vi "Get Log State.vi"(8 "error in (no error)":errorcluster, 10 "Buffer Name (defbuffer1)":string="defbuffer1", 11 "VISA resource name":refnum<visa-resource-name>) -> (0 "error out":errorcluster, 2 "Logging Enabled?":bool, 3 "VISA resource name out":refnum<visa-resource-name>)   [LabVIEW 2022 SP3, in "Keithley 2450.lvlib"]
doc: "This returns whether the reading buffer logs informational events."
uses:
  Keithley 2450.lvlib
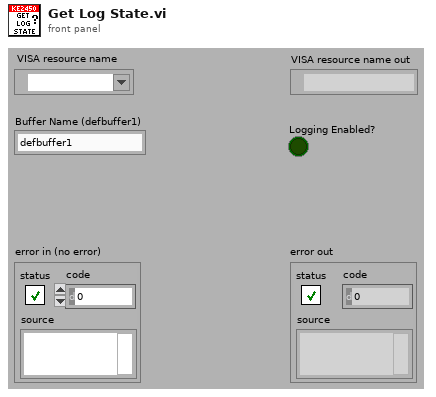
[diagram p1: front panel]
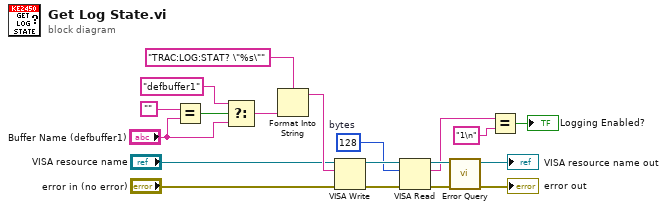
[diagram p0: block diagram]
diagram:
  w4 = u32 128  # bytes
  n1 = Equal?(x="", y="Buffer Name (defbuffer1)") -> (x = y?=w12:bool)
  n2 = Select(t="defbuffer1", s=w12, f="Buffer Name (defbuffer1)") -> (s? t:f=w9:string)
  n3 = Format Into String(format string="TRAC:LOG:STAT? \"%s\"", w9) -> (resulting string=w16:string)  [unwired: 2 in, 1 out]
  n4 = VISA Write(VISA resource name="VISA resource name", write buffer=w16, error in (no error)="error in (no error)") -> (VISA resource name out=w8:refnum<visa-resource-name>, error out=w6:errorcluster)  [unwired: 1 out]
  n5 = VISA Read(VISA resource name=w8, byte count=w4, error in (no error)=w6) -> (VISA resource name out=w7:refnum<visa-resource-name>, read buffer=w1:string, error out=w5:errorcluster)  [unwired: 1 out]
  n6 = call "Error Query.vi"("error in (no error)"=w5, "VISA resource name"=w7) -> ("error out"=→"error out":errorcluster, "VISA resource name out"=→"VISA resource name out":refnum<visa-resource-name>)  [unwired: 8 out]
  n7 = Equal?(x=w1, y="1\n") -> (x = y?=→"Logging Enabled?":bool)
